vi "Error Generator.vi"(8 "error in (no error)":errorcluster, 10 "data return (error code)":u8, 11 "function return":u8(ring) items=["Read Discrete Inputs"=2, "Read Coils"=1, "Write Single Coil"=5, "Write Multiple Coils"=15, "Read Input Register"=4, "Read Holding Registers"=3, "Write Single Register"=6, "Write Multiple Registers"=16, "Read/Write Multiple Registers"=23, "Mask Write Register"=22, "Read FIFO Queue"=24, "Read File Record"=20, "Write File Record"=21, "Read Exception Status"=7, "Diagnostic"=8, "Get Com Event Counter"=11, "Get Com Event Log"=12, "Report Slave ID"=17, "Read Device Identification"=43]) -> (0 "error out":errorcluster)   [LabVIEW 2020, in "SubVIs.lvlib" / "Master Function Definition.lvlib"]
doc: "This VI takes a function error code (>0x80) and its data return and generates a labview error code. The error returned is 900150+Modbus error code."
uses:
  <vilib>/Modbus/subvis/Data and Functions/Master Function Definition/Master Function Definition.lvlib
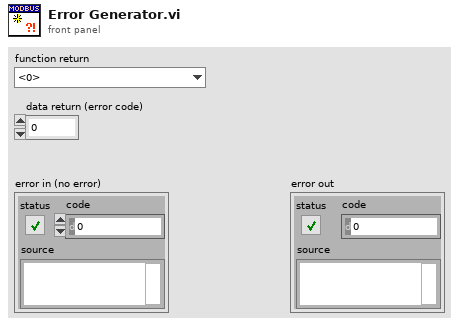
[diagram p1: front panel]
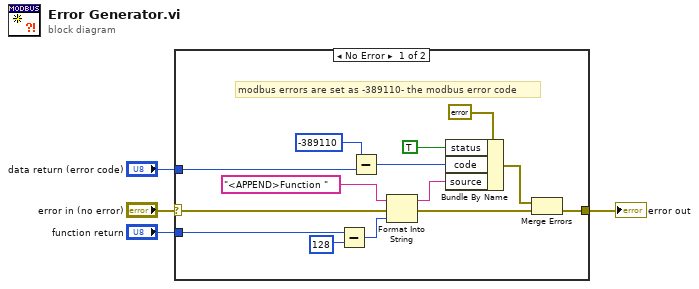
[diagram p0: block diagram]
diagram:
  n1 = case shown="No Error" "error in (no error)" {
    selector: "error in (no error)" -> [w5 w19]
    tunnel: "data return (error code)" -> [w16 _]
    tunnel: "function return" -> [w15 _]
    tunnel: [w10 w19] -> w2
    frame No Error {
      # "modbus errors are set as -389110- the modbus error code"
      n2 = Subtract(x=w15, y=u8 128) -> (x-y=w18:u8)
      n3 = Subtract(x=-389110, y=w16) -> (x-y=w13:i32)
      n4 = Format Into String(initial string="<APPEND>Function " ("format string"), error in=w5, w18) -> (resulting string=w14:string, error out=w6:errorcluster)  [unwired: 1 in]
      n5 = Bundle By Name(cluster=errorcluster {"status"=FALSE, "code"=0, "source"=""} ("error constant"), "status"=TRUE, "code"=w13, "source"=w14) -> (w7:errorcluster)
      n6 = Merge Errors(w7, w6) -> (w10:errorcluster)
    }
    frame Error {
    }
  }
  "error out" <- w2
